vi "Rename_Folder_of_VIs.vi"() -> ()   [LabVIEW 2009]
uses:
  <userlib>/_OpenG.lib/file/file.llb/Build Path - File Names Array__ogtk.vi
  <userlib>/_OpenG.lib/file/file.llb/Strip Path Extension - String__ogtk.vi
  <userlib>/_OpenG.lib/file/file.llb/Strip Path Extension - Path__ogtk.vi
  <userlib>/_OpenG.lib/comparison/comparison.llb/I32 Changed__ogtk.vi
  <userlib>/_OpenG.lib/file/file.llb/Valid Path - Traditional__ogtk.vi
  <userlib>/_OpenG.lib/comparison/comparison.llb/Variant Changed__ogtk.vi
  <userlib>/_OpenG.lib/file/file.llb/Strip Path Extension - 1D Array of Strings__ogtk.vi
panel:
  in  "Swap":bool
  in  "About":bool
  in  "Source Folder":path caption="Folder"
  in  "Folder or LLB":enum32{"Folder", "LLB"}(radio)
  out "Total Progress":u8(slide) scale=0.0..100.0
  out "Progress":u8(slide) scale=0.0..100.0
  in  "Prefix or Suffix":enum32{"Prefix", "Suffix"}(radio)
  in  "Exit Button":bool
  in  "Rename Button":bool
  in  "Recursive":bool
  in  "New Prefix":string caption="New Prefix (\"\": remove existing prefix)"
  in  "Existing Prefix":string caption="Existing Prefix (\"\": prepend new prefix)"
  # "Options"
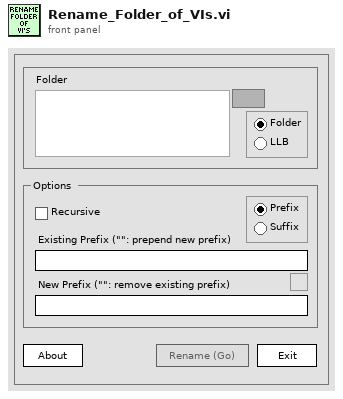
[diagram p1: front panel]
types:
  T1 = cluster{"Version":string, "Build Number":u32, "Build Date/Time":dbl}
  T2 = enum8{"Enabled", "Disabled", "Disabled and Grayed Out"}
  T3 = enum32{"invalid VI type", "Standard VI", "Control VI", "Global VI", "Polymorphic VI", "Configuration VI"}
  T4 = enum32{"invalid VI type", "Standard VI", "Control VI", "Global VI", "Polymorphic VI", "Configuration VI", "SubSystem", "Facade VI", "Method VI", "Statechart Diagram VI"}
  T5 = cluster{"Prompt":string, "Match Pattern":string, "Mode":u32, "Start Path":path}
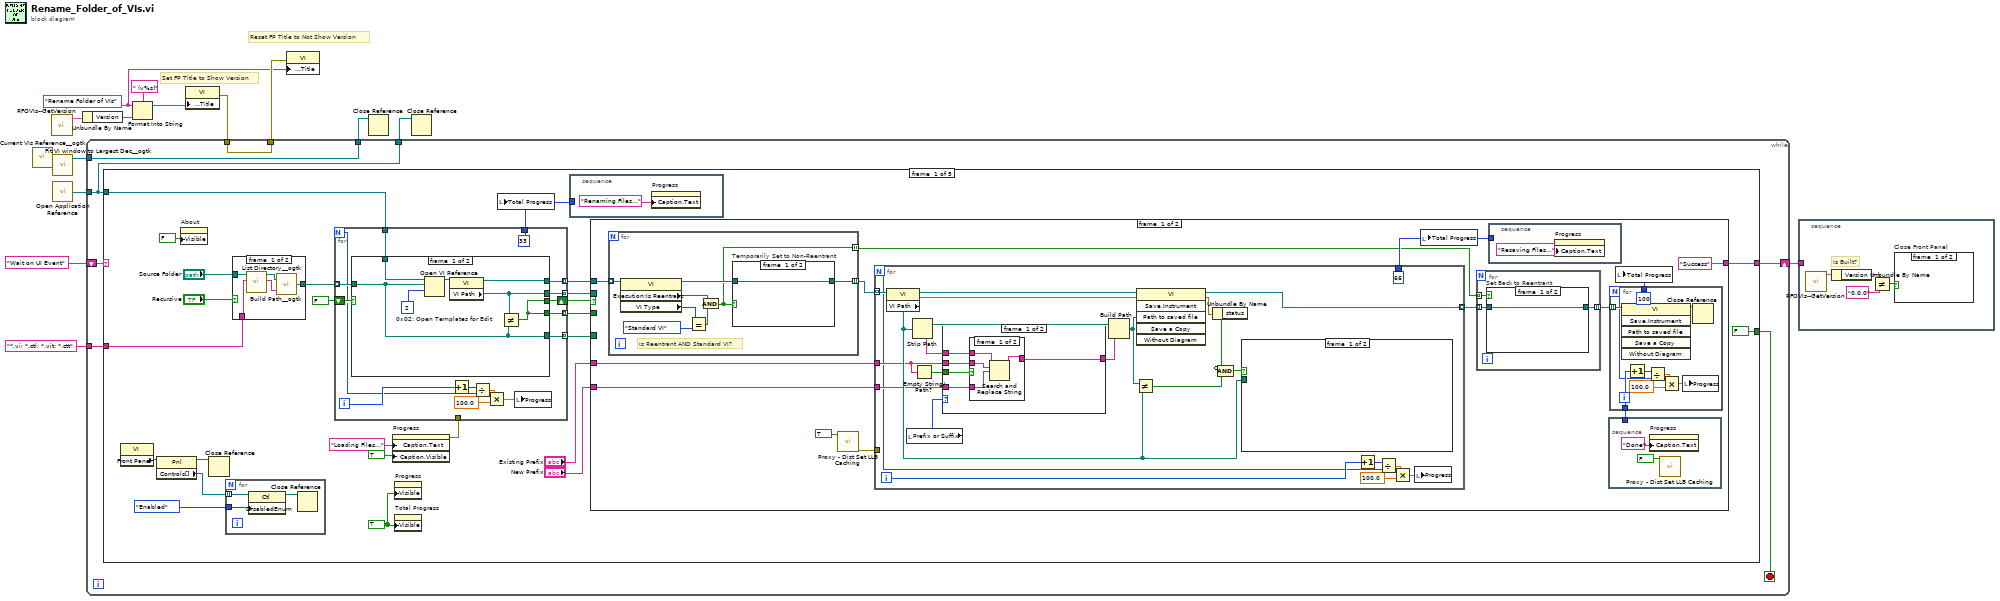
[diagram p0: block diagram]
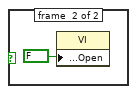
[diagram p2: hidden frame]
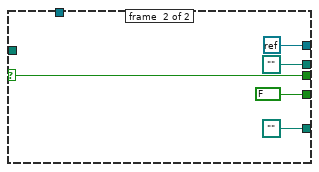
[diagram p3: hidden frame]
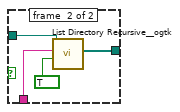
[diagram p4: hidden frame]
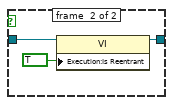
[diagram p5: hidden frame]
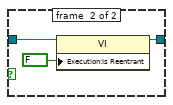
[diagram p6: hidden frame]
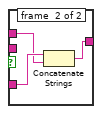
[diagram p7: hidden frame]
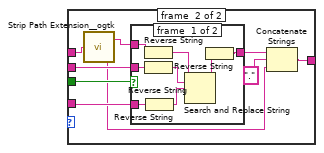
[diagram p8: hidden frame]
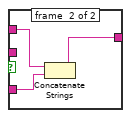
[diagram p9: hidden frame]
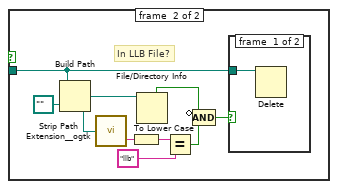
[diagram p10: hidden frame]
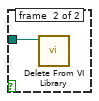
[diagram p11: hidden frame]
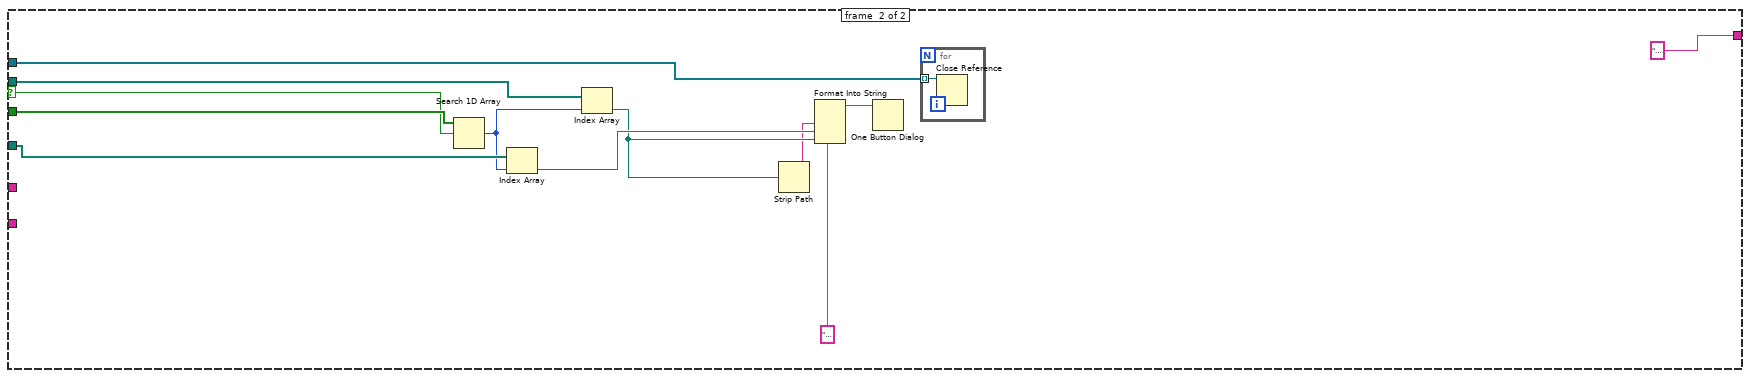
[diagram p12: hidden frame]
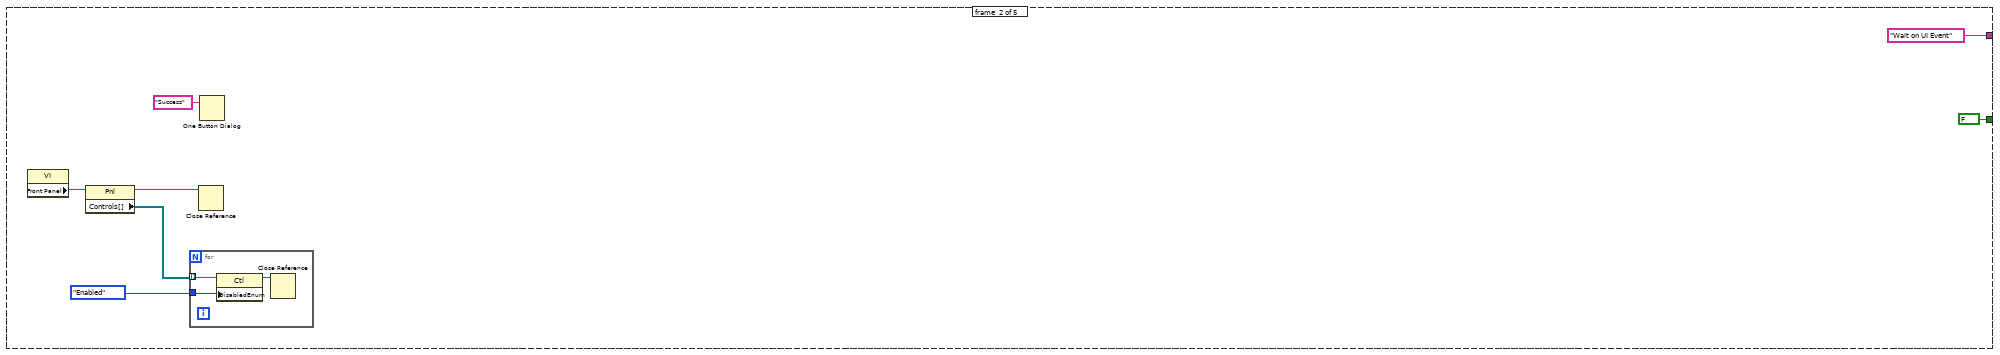
[diagram p13: hidden frame]
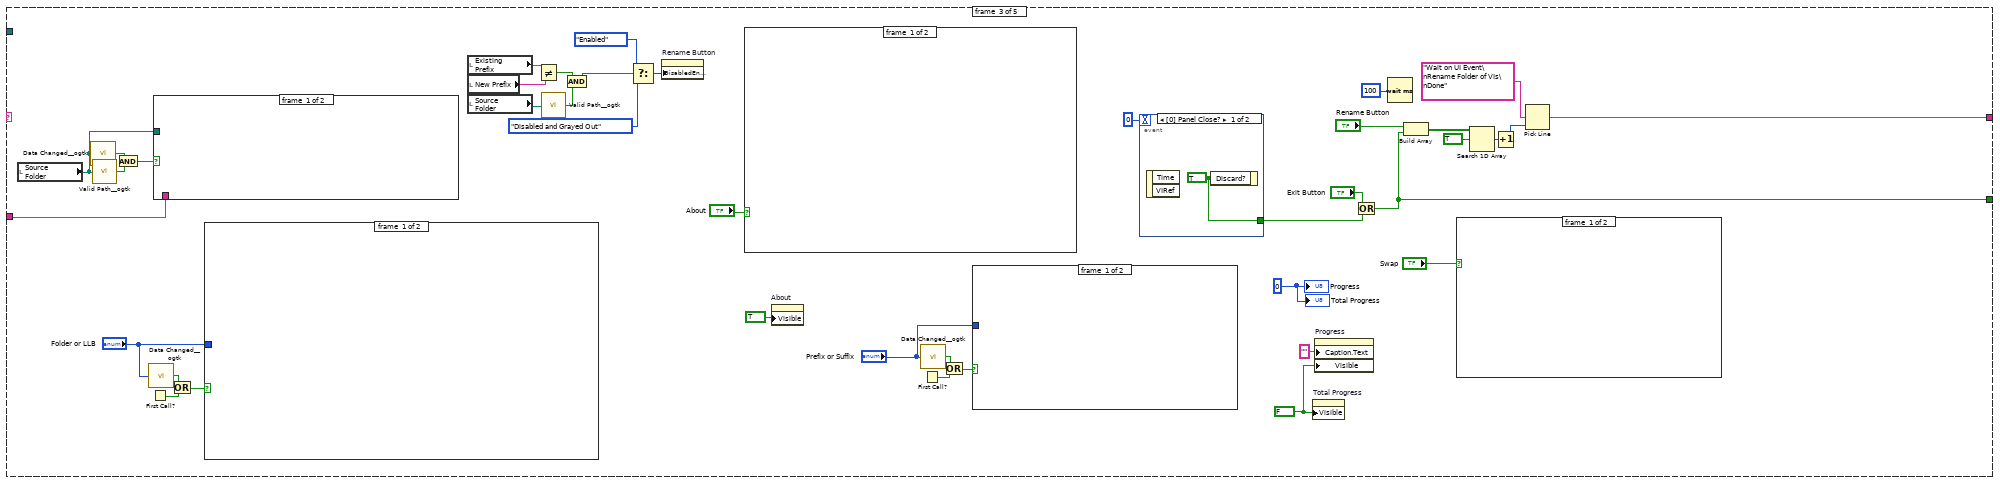
[diagram p14: hidden frame]
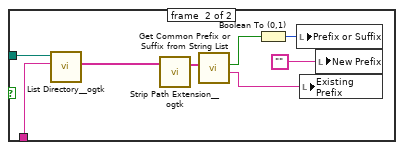
[diagram p15: hidden frame]
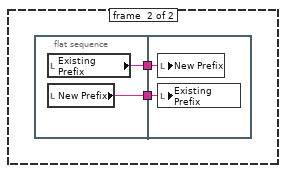
[diagram p16: hidden frame]
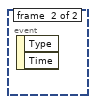
[diagram p17: hidden frame]
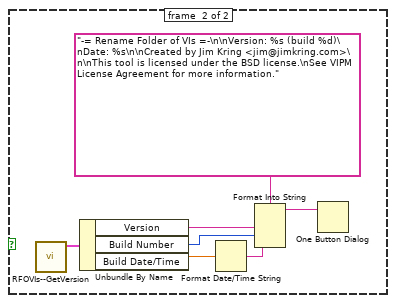
[diagram p18: hidden frame]
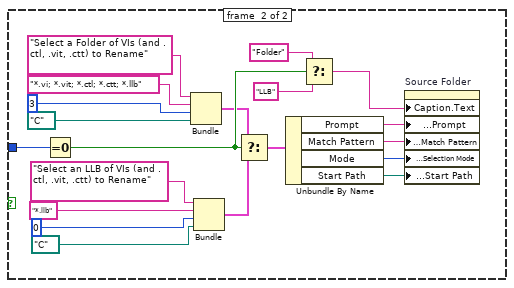
[diagram p19: hidden frame]
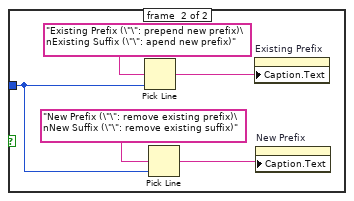
[diagram p20: hidden frame]
diagram:
  w6 = "Rename Folder of VIs" ("format string")
  # "Set FP Title to Show Version"
  # "Reset FP Title to Not Show Version"
  n1 = call <userlib>:"Current VIs Reference__ogtk.vi"() -> ("Current VI's reference"=w14:refnum<vi>)  [unwired: 5 in]
  n2 = call "RFOVIs--GetVersion.vi"() -> ("Version Info"=w12:T1)  [unwired: 10 in, 1 out]
  n3 = call <userlib>:"Fit VI window to Largest Dec__ogtk.vi"("VI Ref (calling VI)"=w14) -> ("dup VI Ref"=w13:refnum<vi>)  [unwired: 5 in, 1 out]
  n4 = call "Open Application Reference.vi"() -> ("application reference"=w3:refnum<vi>)
  n5 = Unbundle By Name(w12) -> ("Version"=w11:string)
  n6 = Format Into String(format string=" (v%s)", initial string=w6, w11) -> (resulting string=w9:string)  [unwired: 1 in, 1 out]
  n7 = property class="VI"("Front Panel Window:Title"=w9) -> (error out=w7:errorcluster)  [unwired: 2 in, 1 out]
  n8 = while {
    tunnel: w13 -> [w18]
    shift-left: "Wait on UI Event" -> [w22]
    shift-right: [w20] -> w5
    tunnel: [w19] -> w8
    tunnel: w7 -> [w19]
    tunnel: [w18] -> w4
    tunnel: w3 -> [w17]
    tunnel: [w17] -> w2
    tunnel: "*.vi; *.ctl; *.vit; *.ctt" ("pattern") -> [w16]
    stop <- w21 stop-if-true
    n9 = case shown="\"Wait on UI Event\"" w22 {
      selector: w22 -> [_ _ _ w313 _]
      tunnel: [FALSE ("Cancel") FALSE ("Cancel") w239 FALSE ("Cancel") TRUE ("Cancel")] -> w21
      tunnel: [w23 "Wait on UI Event" ("pattern") w249 "Wait on UI Event" ("pattern") "" ("pattern")] -> w20
      tunnel: w17 -> [w29 _ _ _ _]
      tunnel: w16 -> [w25 _ w226 _ _]
      frame #0 {
        w31 = TRUE ("Visible")
        n10 = property class="VI"() -> ("Front Panel"=w36:refnum<vi>)  [unwired: 2 in, 2 out]
        n11 = property class="Pnl"(reference=w36) -> (reference out=w34:refnum<vi>, "Controls[]"=w35:refnum<vi>[])  [unwired: 1 in, 1 out]
        n12 = property on="About" class="Boolean"("Visible"=FALSE) -> ()  [unwired: 2 in, 2 out]
        n13 = Close Reference(reference=w34) -> ()  [unwired: 1 in, 1 out]
        n14 = for {
          tunnel: w35 -> [w51] mode=indexing
          tunnel: T2."Enabled" ("Disabled") -> [w49]
          n15 = property on="Property Node" class="Ctl"(reference=w51, "DisabledEnum"=w49) -> (reference out=w50:refnum<vi>)  [unwired: 1 in, 1 out]
          n16 = Close Reference(reference=w50) -> ()  [unwired: 1 in, 1 out]
        }
        n17 = case shown="False" "Recursive" {
          tunnel: "Source Folder" -> [w83 w87]
          tunnel: [w79 w86] -> w40
          tunnel: w25 -> [w82 w85]
          frame #0 {
            n18 = call <userlib>:"List Directory__ogtk.vi"("pattern"=w82, "directory path"=w83) -> ("file names"=w80:string[], "dup directory path"=w81:path)  [unwired: 2 in, 2 out]
            n19 = call-poly <userlib>:"Build Path__ogtk.vi"("name or relative path"=w80, "base path"=w81) -> ("appended path"=w79:path[])
          }
          frame #1 {
            n20 = call <userlib>:"List Directory Recursive__ogtk.vi"("Treat llb files as directories? (FALSE)"=TRUE, "pattern"=w85, "Path"=w87) -> ("file paths"=w86:path[])  [unwired: 5 in, 3 out]
          }
        }
        n21 = property on="Progress" class="Slide (strict)"("Caption.Text"="Loading Files...", "Caption.Visible"=TRUE) -> (error out=w27:errorcluster)  [unwired: 2 in, 1 out]
        n22 = for {
          N -> [w54]
          tunnel: w40 -> [w65] mode=indexing
          tunnel: [w66] -> w41 mode=indexing
          shift-right: [w64] -> w44
          shift-left: FALSE -> [w63]
          tunnel: [w62] -> w45 mode=indexing
          tunnel: [w61] -> w46 mode=indexing
          tunnel: [w60] -> w47 mode=indexing
          tunnel: [u8 33 ("Total Progress")] -> w32
          tunnel: w29 -> [w52]
          tunnel: w27 -> [_]
          i -> [w55]
          n23 = case shown="False" w63 {
            selector: w63 -> [_ w78]
            tunnel: [w72 refnum<k0> refnum] -> w66
            tunnel: w65 -> [w69 _]
            tunnel: [w71 w78] -> w64
            tunnel: [w71 FALSE] -> w62
            tunnel: [w69 path ""] -> w61
            tunnel: [w70 path "" ("Path")] -> w60
            tunnel: w52 -> [w67 _]
            frame #0 {
              w68 = 2  # 0x02: Open Templates for Edit
              n24 = Open VI Reference(application reference (local)=w67, vi path=w69, options=w68) -> (vi reference=w73:refnum<vi>)  [unwired: 3 in, 1 out]
              n25 = property class="VI"(reference=w73) -> (reference out=w72:refnum<vi>, "VI Path"=w70:path)  [unwired: 1 in, 1 out]
              n26 = Not Equal?(x=w70, y=w69) -> (x != y?=w71:bool)
            }
            frame #1 {
            }
          }
          n27 = Increment(x=w55) -> (x+1=w56:i32)
          n28 = Divide(x=w56, y=w54) -> (x/y=w58:dbl)
          n29 = Multiply(x=w58, y=100.0) -> (x*y=w59:dbl)
          n30 = local write "Progress"(w59) -> ()
        }
        n31 = property on="Progress" class="Slide (strict)"("Visible"=w31) -> ()  [unwired: 2 in, 2 out]
        n32 = property on="Total Progress" class="Slide (strict)"("Visible"=w31) -> ()  [unwired: 2 in, 2 out]
        n33 = local write "Total Progress"(w32) -> ()
        n34 = stacked-sequence {
          tunnel: w32 -> [_]
          frame #0 {
            n35 = property on="Progress" class="Slide (strict)"("Caption.Text"="Renaming Files...") -> ()  [unwired: 2 in, 2 out]
          }
        }
        n36 = case shown="False" w44 {
          selector: w44 -> [_ w209]
          tunnel: "Existing Prefix" -> [w100 _]
          tunnel: "New Prefix" -> [w99 _]
          tunnel: w41 -> [w94 w208]
          tunnel: w45 -> [_ w210]
          tunnel: w46 -> [_ w207]
          tunnel: w47 -> [_ w206]
          tunnel: ["Success" ("pattern") "Wait on UI Event" ("pattern")] -> w23
          frame #0 {
            n37 = for {
              tunnel: w94 -> [w115] mode=indexing
              tunnel: [w109] -> w90 mode=indexing
              tunnel: [w108] -> w93 mode=indexing
              # "Is Reentrant AND Standard VI?"
              n38 = property class="VI"(reference=w115) -> (reference out=w110:refnum<vi>, "Execution:Is Reentrant"=w111:bool, "VI Type"=w113:T4)  [unwired: 1 in, 1 out]
              n39 = Equal?(x=w113, y=T3."Standard VI" ("VI Type")) -> (x = y?=w112:bool)
              n40 = And(x=w111, y=w112) -> (x .and. y?=w109:bool)
              n41 = case "Temporarily Set to Non-Reentrant" shown="True" w109 {
                tunnel: w110 -> [w116 w119]
                tunnel: [w116 w117] -> w108
                frame #0 {
                }
                frame #1 {
                  n42 = property class="VI"(reference=w119, "Execution:Is Reentrant"=FALSE) -> (reference out=w117:refnum<vi>)  [unwired: 1 in, 1 out]
                }
              }
            }
            n43 = call "Proxy - Dist Set LLB Caching.vi"("enable?"=TRUE) -> ("error out"=w88:errorcluster)  [unwired: 10 in]
            n44 = for {
              N -> [w134]
              tunnel: w100 -> [w145]
              tunnel: w99 -> [w146]
              tunnel: w93 -> [w143] mode=indexing
              tunnel: [w141] -> w92 mode=indexing
              tunnel: [u8 66 ("Total Progress")] -> w97
              tunnel: w88 -> [_]
              i -> [w135]
              n45 = property class="VI"(reference=w143) -> (reference out=w152:refnum<vi>, error out=w151:errorcluster, "VI Path"=w147:path)  [unwired: 1 in]
              n46 = local read "Prefix or Suffix"() -> (w140:enum32{"Prefix", "Suffix"})
              n47 = Strip Path(path=w147) -> (stripped path=w155:path, name=w154:string)
              n48 = Empty String/Path?(string/path=w145) -> (empty?=w144:bool)
              n49 = case shown="\"Prefix\", Default" w140 {
                tunnel: w154 -> [w160 w176]
                tunnel: [w159 w168] -> w153
                tunnel: w146 -> [w158 w173]
                tunnel: w145 -> [w157 w172]
                tunnel: w144 -> [w156 w175]
                frame #0 {
                  n50 = case shown="True" w156 {
                    tunnel: w160 -> [w164 w166]
                    tunnel: [w163 w165] -> w159
                    tunnel: w158 -> [w162 w167]
                    tunnel: w157 -> [w161 _]
                    frame #0 {
                      n51 = Search and Replace String(input string=w164, search string=w161, replace string=w162) -> (result string=w163:string)  [unwired: 5 in, 3 out]
                    }
                    frame #1 {
                      n52 = Concatenate Strings(w167, w166) -> (w165:string)
                    }
                  }
                }
                frame #1 {
                  n53 = call-poly <userlib>:"Strip Path Extension__ogtk.vi"("path"=w176) -> ("root"=w174:string, "extension"=w169:string)
                  n54 = case shown="False" w175 {
                    tunnel: [w180 w187] -> w170
                    tunnel: w173 -> [w183 w185]
                    tunnel: w174 -> [w177 w186]
                    tunnel: w172 -> [w184 _]
                    frame #0 {
                      n55 = Reverse String(1:w177) -> (0:w178:string)
                      n56 = Reverse String(1:w184) -> (0:w182:string)
                      n57 = Reverse String(1:w183) -> (0:w181:string)
                      n58 = Search and Replace String(input string=w178, search string=w182, replace string=w181) -> (result string=w179:string)  [unwired: 5 in, 3 out]
                      n59 = Reverse String(1:w179) -> (0:w180:string)
                    }
                    frame #1 {
                      n60 = Concatenate Strings(w186, w185) -> (w187:string)
                    }
                  }
                  n61 = Concatenate Strings(w170, "." ("Substring"), w169) -> (w168:string)
                }
              }
              n62 = Build Path(base path=w155, name or relative path=w153) -> (appended path=w150:path)
              n63 = Not Equal?(x=w150, y=w147) -> (x != y?=w149:bool)
              n64 = invoke class="VI" method="Save.Instrument"(reference=w152, error in=w151, "Path to saved file"=w150) -> (reference out=w141:refnum<vi>, error out=w142:errorcluster)  [unwired: 3 in, 4 out]
              n65 = Unbundle By Name(w142) -> ("status"=w132:bool)
              n66 = Compound Arithmetic op=AND(invert w132, w149) -> (w148:bool)
              n67 = case shown="True" w148 {
                tunnel: w147 -> [_ w188]
                frame #0 {
                }
                frame #1 {
                  # "In LLB File?"
                  n68 = Build Path(base path=w188, name or relative path=path ".." ("base path")) -> (appended path=w195:path)
                  n69 = call-poly <userlib>:"Strip Path Extension__ogtk.vi"("path"=w195) -> ("extension"=w194:string)  [unwired: 1 out]
                  n70 = To Lower Case(string=w194) -> (all lower case string=w193:string)
                  n71 = File/Directory Info(path=w195) -> (directory=w191:bool)  [unwired: 1 in, 6 out]
                  n72 = Equal?(x=w193, y="llb" ("all lower case string")) -> (x = y?=w190:bool)
                  n73 = Compound Arithmetic op=AND(invert w191, w190) -> (w189:bool)
                  n74 = case shown="True" w189 {
                    tunnel: w188 -> [w197 w198]
                    frame #0 {
                      n75 = Delete(path (use dialog)=w197) -> ()  [unwired: 4 in, 3 out]
                    }
                    frame #1 {
                      n76 = call <vilib>:"Delete From VI Library.vi"("path"=w198) -> ()  [unwired: 10 in, 1 out]
                    }
                  }
                }
              }
              n77 = Increment(x=w135) -> (x+1=w136:i32)
              n78 = Divide(x=w136, y=w134) -> (x/y=w138:dbl)
              n79 = Multiply(x=w138, y=100.0) -> (x*y=w139:dbl)
              n80 = local write "Progress"(w139) -> ()
            }
            n81 = local write "Total Progress"(w97) -> ()
            n82 = for {
              tunnel: [w103] -> w91 mode=indexing
              tunnel: w92 -> [w102] mode=indexing
              tunnel: w90 -> [w101] mode=indexing
              n83 = case "Set Back to Reentrant" shown="True" w101 {
                tunnel: w102 -> [w104 w107]
                tunnel: [w104 w105] -> w103
                frame #0 {
                }
                frame #1 {
                  n84 = property class="VI"(reference=w107, "Execution:Is Reentrant"=TRUE) -> (reference out=w105:refnum<vi>)  [unwired: 1 in, 1 out]
                }
              }
            }
            n85 = stacked-sequence {
              tunnel: w97 -> [_]
              frame #0 {
                n86 = property on="Progress" class="Slide (strict)"("Caption.Text"="Resaving Files...") -> ()  [unwired: 2 in, 2 out]
              }
            }
            n87 = for {
              N -> [w124]
              tunnel: w91 -> [w131] mode=indexing
              tunnel: [u8 100 ("Total Progress")] -> w96
              tunnel: [w125] -> w95
              i -> [w125]
              n88 = invoke class="VI" method="Save.Instrument"(reference=w131) -> (reference out=w130:refnum<vi>)  [unwired: 5 in, 5 out]
              n89 = Increment(x=w125) -> (x+1=w126:i32)
              n90 = Divide(x=w126, y=w124) -> (x/y=w128:dbl)
              n91 = Multiply(x=w128, y=100.0) -> (x*y=w129:dbl)
              n92 = local write "Progress"(w129) -> ()
              n93 = Close Reference(reference=w130) -> ()  [unwired: 1 in, 1 out]
            }
            n94 = stacked-sequence {
              tunnel: w95 -> [_]
              frame #0 {
                n95 = property on="Progress" class="Slide (strict)"("Caption.Text"="Done") -> ()  [unwired: 2 in, 2 out]
                n96 = call "Proxy - Dist Set LLB Caching.vi"("enable?"=FALSE) -> ()  [unwired: 10 in, 1 out]
              }
            }
            n97 = local write "Total Progress"(w96) -> ()
          }
          frame #1 {
            n98 = Search 1D Array(1D array=w210, element=w209) -> (index of element=w205:i32)  [unwired: 1 in]
            n99 = Index Array(array=w207, index=w205) -> (element=w204:path)
            n100 = Index Array(array=w206, index=w205) -> (element=w203:path)
            n101 = Strip Path(path=w203) -> (name=w202:string)  [unwired: 1 out]
            n102 = Format Into String(format string="Cannot rename folder. \"%s\" expected in the following location:\n\n%s\n\nfound already in memory at:\n\n%s\n\nNo VIs renamed.", w202, w204, w203) -> (resulting string=w201:string)  [unwired: 2 in, 1 out]
            n103 = One Button Dialog(message=w201) -> ()  [unwired: 1 in, 1 out]
            n104 = for {
              tunnel: w208 -> [w211] mode=indexing
              n105 = Close Reference(reference=w211) -> ()  [unwired: 1 in, 1 out]
            }
          }
        }
      }
      frame #1 {
        n106 = property class="VI"() -> ("Front Panel"=w216:refnum<vi>)  [unwired: 2 in, 2 out]
        n107 = property class="Pnl"(reference=w216) -> (reference out=w214:refnum<vi>, "Controls[]"=w215:refnum<vi>[])  [unwired: 1 in, 1 out]
        n108 = for {
          tunnel: w215 -> [w221] mode=indexing
          tunnel: T2."Enabled" ("Disabled") -> [w219]
          n109 = property on="Property Node" class="Ctl"(reference=w221, "DisabledEnum"=w219) -> (reference out=w220:refnum<vi>)  [unwired: 1 in, 1 out]
          n110 = Close Reference(reference=w220) -> ()  [unwired: 1 in, 1 out]
        }
        n111 = Close Reference(reference=w214) -> ()  [unwired: 1 in, 1 out]
        n112 = One Button Dialog(message="Success") -> ()  [unwired: 1 in, 1 out]
      }
      frame #2 {
        w247 = FALSE ("Visible")
        w248 = u8 0 ("Progress")
        n113 = local read "Source Folder"() -> (w225:path)
        n114 = call-poly <userlib>:"Data Changed__ogtk.vi"("Variant"=w225) -> ("Changed"=w229:bool)
        n115 = call-poly <userlib>:"Valid Path__ogtk.vi"("path"=w225) -> ("valid"=w228:bool)
        n116 = And(x=w229, y=w228) -> (x .and. y?=w227:bool)
        n117 = First Call?() -> (First Call?: T/F=w244:bool)
        n118 = call-poly <userlib>:"Data Changed__ogtk.vi"("I32"="Folder or LLB") -> ("Changed"=w243:bool)
        n119 = case shown="True" w227 {
          tunnel: w225 -> [_ w269]
          tunnel: w226 -> [_ w268]
          frame #0 {
          }
          frame #1 {
            n120 = call <userlib>:"List Directory__ogtk.vi"("pattern"=w268, "directory path"=w269) -> ("file names"=w267:string[])  [unwired: 2 in, 3 out]
            n121 = call-poly <userlib>:"Strip Path Extension__ogtk.vi"("paths"=w267) -> ("roots"=w266:string[])  [unwired: 1 out]
            n122 = call "Get Common Prefix or Suffix from String List.vi"("Strings"=w266) -> ("Common Part"=w264:string, "Suffix? (F: Prefix)"=w263:bool)  [unwired: 9 in]
            n123 = Boolean To (0,1)(Boolean=w263) -> (0, 1=w262:i16)
            n124 = local write "Prefix or Suffix"(w262) -> ()
            n125 = local write "Existing Prefix"(w264) -> ()
            n126 = local write "New Prefix"("") -> ()
          }
        }
        n127 = Or(x=w243, y=w244) -> (x .or. y?=w245:bool)
        n128 = case shown="True" w245 {
          tunnel: "Folder or LLB" -> [_ w302]
          frame #0 {
          }
          frame #1 {
            n129 = Equal To 0?(x=w302) -> (x = 0?=w301:bool)
            n130 = Bundle("Prompt"="Select a Folder of VIs (and .ctl, .vit, .ctt) to Rename", "Match Pattern"="*.vi; *.vit; *.ctl; *.ctt; *.llb", "Mode"=u32 3, "Start Path"=path "C:/") -> (w290:T5)  [unwired: 1 in]
            n131 = Bundle("Prompt"="Select an LLB of VIs (and .ctl, .vit, .ctt) to Rename", "Match Pattern"="*.llb", "Mode"=u32 0, "Start Path"=path "C:/") -> (w291:T5)  [unwired: 1 in]
            n132 = Select(t=w290, s=w301, f=w291) -> (s? t:f=w289:T5)
            n133 = Unbundle By Name(w289) -> ("Prompt"=w288:string, "Match Pattern"=w287:string, "Mode"=w286:u32, "Start Path"=w285:path)
            n134 = Select(t="Folder", s=w301, f="LLB") -> (s? t:f=w284:string)
            n135 = property on="Source Folder" class="Path"("Caption.Text"=w284, "Browse Options:Prompt"=w288, "Browse Options:Match Pattern"=w287, "Browse Options:Selection Mode"=w286, "Browse Options:Start Path"=w285) -> ()  [unwired: 2 in, 2 out]
          }
        }
        n136 = local read "Existing Prefix"() -> (w236:string)
        n137 = local read "New Prefix"() -> (w235:string)
        n138 = local read "Source Folder"() -> (w234:path)
        n139 = Not Equal?(x=w236, y=w235) -> (x != y?=w233:bool)
        n140 = call-poly <userlib>:"Valid Path__ogtk.vi"("path"=w234) -> ("valid"=w232:bool)
        n141 = And(x=w233, y=w232) -> (x .and. y?=w231:bool)
        n142 = Select(t=T2."Enabled" ("Disabled"), s=w231, f=T2."Disabled and Grayed Out" ("Disabled")) -> (s? t:f=w223:T2)
        n143 = property on="Rename Button" class="Boolean"("DisabledEnum"=w223) -> ()  [unwired: 2 in, 2 out]
        n144 = case shown="True" "About" {
          frame #0 {
          }
          frame #1 {
            n145 = call "RFOVIs--GetVersion.vi"() -> ("Version Info"=w282:T1)  [unwired: 10 in, 1 out]
            n146 = Unbundle By Name(w282) -> ("Version"=w281:string, "Build Number"=w280:u32, "Build Date/Time"=w278:dbl)
            n147 = Format Date/Time String(seconds (now)=w278) -> (date/time string=w277:string)  [unwired: 2 in]
            n148 = Format Into String(format string="-= Rename Folder of VIs =-\n\nVersion: %s (build %d)\nDate: %s\n\nCreated by Jim Kring <jim@jimkring.com>\n\nThis tool is licensed under the BSD license.\nSee VIPM License Agreement for more information." ("pattern"), w281, w280, w277) -> (resulting string=w279:string)  [unwired: 2 in, 1 out]
            n149 = One Button Dialog(message=w279) -> ()  [unwired: 1 in, 1 out]
          }
        }
        n150 = property on="About" class="Boolean"("Visible"=TRUE) -> ()  [unwired: 2 in, 2 out]
        n151 = First Call?() -> (First Call?: T/F=w259:bool)
        n152 = call-poly <userlib>:"Data Changed__ogtk.vi"("I32"="Prefix or Suffix") -> ("Changed"=w260:bool)
        n153 = Or(x=w260, y=w259) -> (x .or. y?=w258:bool)
        n154 = case shown="True" w258 {
          tunnel: "Prefix or Suffix" -> [_ w308]
          frame #0 {
          }
          frame #1 {
            n155 = Pick Line(multi-line string="Existing Prefix (\"\": prepend new prefix)\nExisting Suffix (\"\": apend new prefix)", line index=w308) -> (output string=w305:string)  [unwired: 1 in]
            n156 = Pick Line(multi-line string="New Prefix (\"\": remove existing prefix)\nNew Suffix (\"\": remove existing suffix)", line index=w308) -> (output string=w304:string)  [unwired: 1 in]
            n157 = property on="Existing Prefix" class="String"("Caption.Text"=w305) -> ()  [unwired: 2 in, 2 out]
            n158 = property on="New Prefix" class="String"("Caption.Text"=w304) -> ()  [unwired: 2 in, 2 out]
          }
        }
        n159 = event shown="[0] Panel Close?" {
          selector: _ -> [_ _]
          dyn-events: _ -> [_ _]
          timeout: 0 -> [_ _]
          tunnel: [w276 _] -> w240
          event #0 {
            w276 = TRUE ("Discard?")
            n160 = event-data() -> ()  [unwired: 1 in, 2 out]
            n161 = event-data("Discard?"=w276) -> ()  [unwired: 1 in, 1 out]
          }
          event #1 {
            n162 = event-data() -> ()  [unwired: 1 in, 2 out]
          }
        }
        n163 = property on="Total Progress" class="Slide (strict)"("Visible"=w247) -> ()  [unwired: 2 in, 2 out]
        n164 = property on="Progress" class="Slide (strict)"("Caption.Text"="", "Visible"=w247) -> ()  [unwired: 2 in, 2 out]
        n165 = Or(x="Exit Button", y=w240) -> (x .or. y?=w239:bool)
        n166 = Wait (ms)(milliseconds to wait=u32 100) -> ()  [unwired: 1 out]
        n167 = Build Array("Rename Button", w239) -> (w255:bool[])
        n168 = case shown="True" "Swap" {
          frame #0 {
          }
          frame #1 {
            n169 = flat-sequence {
              tunnel: [w273] -> w271
              tunnel: [w272] -> w270
              tunnel: w271 -> [w275]
              tunnel: w270 -> [w274]
              frame #0 {
                n170 = local read "Existing Prefix"() -> (w273:string)
                n171 = local read "New Prefix"() -> (w272:string)
              }
              frame #1 {
                n172 = local write "New Prefix"(w275) -> ()
                n173 = local write "Existing Prefix"(w274) -> ()
              }
            }
          }
        }
        n174 = Search 1D Array(1D array=w255, element=TRUE) -> (index of element=w253:i32)  [unwired: 1 in]
        n175 = Increment(x=w253) -> (x+1=w252:i32)
        n176 = Pick Line(multi-line string="Wait on UI Event\nRename Folder of VIs\nDone" ("pattern"), line index=w252) -> (output string=w249:string)  [unwired: 1 in]
        "Total Progress" <- w248
        "Progress" <- w248
      }
      frame #3 {
        n177 = Format Into String(format string="Error Undefined Software State \"%s\"", w313) -> (resulting string=w310:string)  [unwired: 2 in, 1 out]
        n178 = One Button Dialog(message=w310) -> ()  [unwired: 1 in, 1 out]
      }
      frame #4 {
      }
    }
  }
  n179 = property class="VI"(error in=w8, "Front Panel Window:Title"=w6) -> ()  [unwired: 1 in, 2 out]
  n180 = Close Reference(reference=w4) -> ()  [unwired: 1 in, 1 out]
  n181 = Close Reference(reference=w2) -> ()  [unwired: 1 in, 1 out]
  n182 = stacked-sequence {
    tunnel: w5 -> [_]
    frame #0 {
      # "Is Built?"
      n183 = call "RFOVIs--GetVersion.vi"() -> ("Version Info"=w319:T1)  [unwired: 10 in, 1 out]
      n184 = Unbundle By Name(w319) -> ("Version"=w318:string)
      n185 = Not Equal?(x=w318, y="0.0.0" ("Version")) -> (x != y?=w316:bool)
      n186 = case "Close Front Panel" shown="True" w316 {
        frame #0 {
        }
        frame #1 {
          n187 = property class="VI"("Front Panel Window:Open"=FALSE) -> ()  [unwired: 2 in, 2 out]
        }
      }
    }
  }
